vi "SetButtonDefinitionFile.vi"(8 "ErrorIn":errorcluster, 10 "ButtonDefinitionFile":string, 11 "ReferenceIn":refnum<class "VerticalButtonBar.lvclass">) -> (0 "ErrorOut":errorcluster, 3 "ReferenceIn":refnum<class "VerticalButtonBar.lvclass">)   [LabVIEW 2021, in "VerticalButtonBar.lvclass"]
uses:
  VerticalButtonBar.lvclass
  ButtonCollection/ButtonCollection.lvclass
  VerticalButtonBar.lvclass/VerticalButtonBar.ctl
  Library_TAF_ApplicationFramework/Application/Application.lvclass
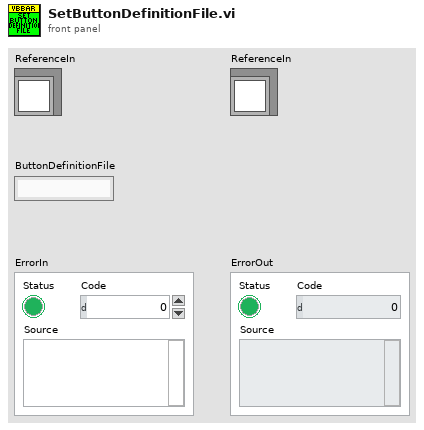
[diagram p1: front panel]
types:
  T1 = typedef "VerticalButtonBar.lvclass/ObjectAttributes.ctl" = cluster{"Interfaces":cluster{"IDockGUI":refnum<class "IDockGUI.lvclass">, "Authorizer":refnum<class "IAuthorization.lvclass">}, "Locals":cluster{"ButtonBar":refnum<class "ButtonCollection.lvclass">, "BaseConfigurationPath":path, "Labels":cluster{"Label":string, "Value":string}[]}, "Persistent":cluster{"ButtonDefinitionFile":string}}
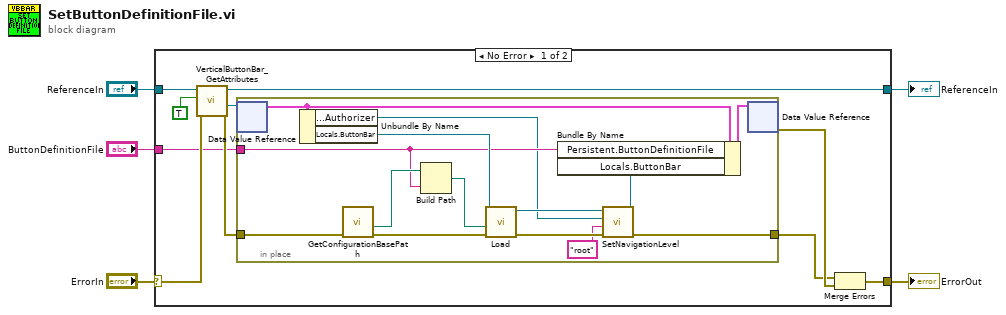
[diagram p0: block diagram]
diagram:
  n1 = case shown="No Error" "ErrorIn" {
    selector: "ErrorIn" -> [w15 w31]
    tunnel: [w13 w31] -> w4
    tunnel: [w9 w30] -> w2
    tunnel: "ReferenceIn" -> [w10 w30]
    tunnel: "ButtonDefinitionFile" -> [w6 _]
    frame No Error {
      n2 = call "VerticalButtonBar_GetAttributes.vi"("ErrorIn"=w15, "OnlyGetDvrReference(False)"=TRUE, "ReferenceIn"=w10) -> ("ErrorOut"=w12:errorcluster, "DataRef"=w7:refnum<data-value>, "ReferenceOut"=w9:refnum<class "VerticalButtonBar.lvclass">)  [unwired: 5 in, 1 out]
      n3 = in-place {
        in-place-border: w6 -> [w19]
        in-place-border: w12 -> [w28]
        in-place-border: [w29] -> w11
        n4 = in-place-dvr #1(w7) -> (w24:T1)  [unwired: 1 out]
        n5 = Unbundle By Name(w24) -> ("Interfaces.Authorizer"=w16:refnum<class "IAuthorization.lvclass">, "Locals.ButtonBar"=w23:refnum<class "ButtonCollection.lvclass">)
        n6 = call "GetConfigurationBasePath.vi"("ErrorIn"=w28) -> ("ErrorOut"=w27:errorcluster, "BasePath"=w20:path)  [unwired: 9 in]
        n7 = Build Path(base path=w20, name or relative path=w19) -> (appended path=w18:path)
        n8 = call "Load.vi"("ErrorIn"=w27, "Path"=w18, "ObjectIn"=w23) -> ("ErrorOut"=w26:errorcluster, "ObjectOut"=w17:refnum<class "ButtonCollection.lvclass">)  [unwired: 7 in]
        n9 = call-dynamic "SetNavigationLevel.vi"("ErrorIn"=w26, "NavigationName"="root", "Authorization"=w16, "ObjectIn"=w17) -> ("ErrorOut"=w29:errorcluster, "ObjectOut"=w21:refnum<class "ButtonCollection.lvclass">)  [unwired: 6 in]
        n10 = Bundle By Name(cluster=w24, "Persistent.ButtonDefinitionFile"=w19, "Locals.ButtonBar"=w21) -> (w25:T1)
        n11 = in-place-dvr #1(w25) -> (w14:errorcluster)  [unwired: 1 out]
      }
      n12 = Merge Errors(w11, w14) -> (w13:errorcluster)
    }
    frame Error {
    }
  }
  "ErrorOut" <- w4
  "ReferenceIn" <- w2
